vi "BusBase_Create.vi"(8 "Error In":errorcluster, 11 "reference in":refnum<class "BusBase.lvclass">) -> (0 "Error Out":errorcluster, 3 "reference out":refnum<class "BusBase.lvclass">)   [LabVIEW 2021, in "BusBase.lvlib" / "BusBase.lvclass"]
uses:
  BusBase.lvclass
  C:/Localdata/Projects/TriekselSoft/TriekselsoftApplicationFramework/Source/.Externals/Library_TAF_ApplicationFramework/TAFBaseGUI/TAFBaseGUI.lvclass
  Library_TAF_ApplicationFramework/TAFBaseGUI/TAFBaseGUI.lvclass
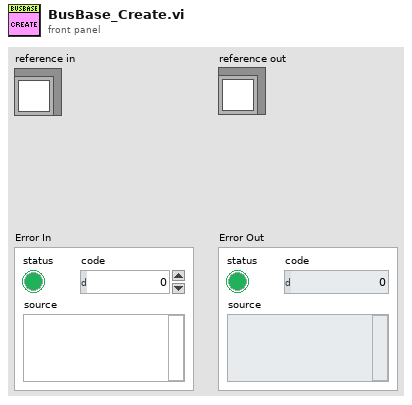
[diagram p1: front panel]
types:
  T1 = typedef "BusBase.lvlib/BusBase.lvclass/ObjectAttributes.ctl" = cluster{"Interfaces":cluster{"TargetClasses":refnum<class>[]}, "Locals":cluster{"MainGUIActive":refnum<queue>}, "Persistent":cluster{"Dummy":bool}}
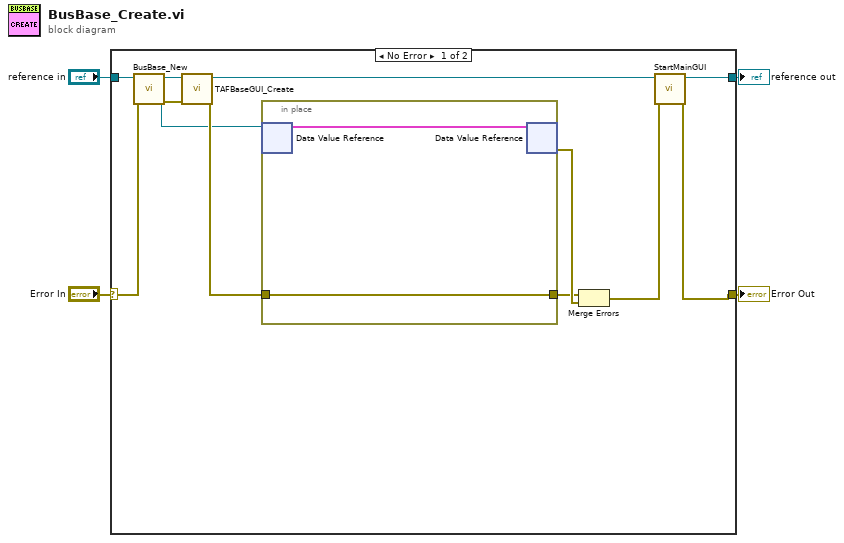
[diagram p0: block diagram]
diagram:
  n1 = case shown="No Error" "Error In" {
    selector: "Error In" -> [w12 w20]
    tunnel: [w5 w20] -> w3
    tunnel: "reference in" -> [w13 w19]
    tunnel: [w7 w19] -> w1
    frame No Error {
      n2 = call "BusBase_New.vi"("error in (no error)"=w12, "reference in"=w13) -> ("error out"=w10:errorcluster, "DVRRefOut"=w9:refnum<data-value>, "reference out"=w11:refnum<class "BusBase.lvclass">)  [unwired: 6 in, 1 out]
      n3 = call "TAFBaseGUI_Create.vi"("Error In"=w10, "reference in"=w11) -> ("Error Out"=w15:errorcluster, "reference out"=w8:refnum<class "BusBase.lvclass">)  [unwired: 8 in]
      n4 = in-place {
        in-place-border: w15 -> [w18]
        in-place-border: [w18] -> w14
        n5 = in-place-dvr #1(w9) -> (w17:T1)  [unwired: 1 out]
        n6 = in-place-dvr #1(w17) -> (w16:errorcluster)  [unwired: 1 out]
      }
      n7 = Merge Errors(w14, w16) -> (w6:errorcluster)
      n8 = call "StartMainGUI.vi"("Error In"=w6, "reference in"=w8) -> ("Error Out"=w5:errorcluster, "reference out"=w7:refnum<class "BusBase.lvclass">)  [unwired: 6 in, 2 out]
    }
    frame Error {
      # "VI-TechBaseTemplate_Simple_4x4x4"
    }
  }
  "Error Out" <- w3
  "reference out" <- w1
